vi "Fringe Scan.vi"() -> ()   [LabVIEW 2010]
uses:
  <instrlib>/Keithley 27XX/Public/Data/Read Multiple Direct.vi
  <instrlib>/Keithley 27XX/Keithley 27XX.lvlib
  <vilib>/Analysis/NI_AALBase.lvlib
panel:
  out "Last Value, Volts":dbl
  out "Midpoint":dbl format="%0.3f"
  out "Vpp":dbl
  in  "Integration Time":u16(ring)=10 items=["Slow"=50, "Medium"=10, "Fast"=1]
  out "Waveform Chart":dbl[](graph)
  in  "stop":bool
  in  "VISA resource name":refnum<visa-resource-name>="GPIB0::17::INSTR"
  in  "Serial Configuration (Delicate)":T1={"Baud Rate (9600)"=9600, "Flow Control (1: XON/XOFF)"=1, "Termination Char (0:CR)"=0} {"Termination Char (0:CR)" items=["CR", "LF"]; "Flow Control (1: XON/XOFF)" items=["None", "XON/XOFF", "RTS/CTS (2701 Only)", "XON/XOFF & RTS/CTS (2701 Only)"]; "Baud Rate (9600)" items=["300"=300, "600"=600, "1200"=1200, "2400"=2400, "4800"=4800, "9600"=9600, "19.2k"=19200, "38.4k (2701 Only)"=38400, "57.6k (2701 Only)"=57600, "115.2k (2701 Only)"=115200]}
  # "For use with Keithley 2700, default GPIB address 17"
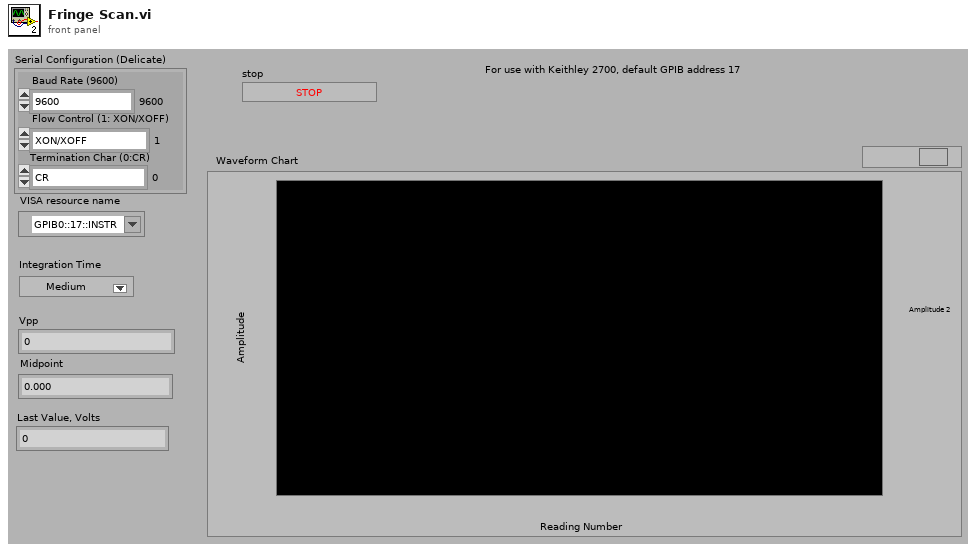
[diagram p1: front panel]
types:
  T1 = cluster{"Baud Rate (9600)":u32, "Flow Control (1: XON/XOFF)":u16, "Termination Char (0:CR)":u16}
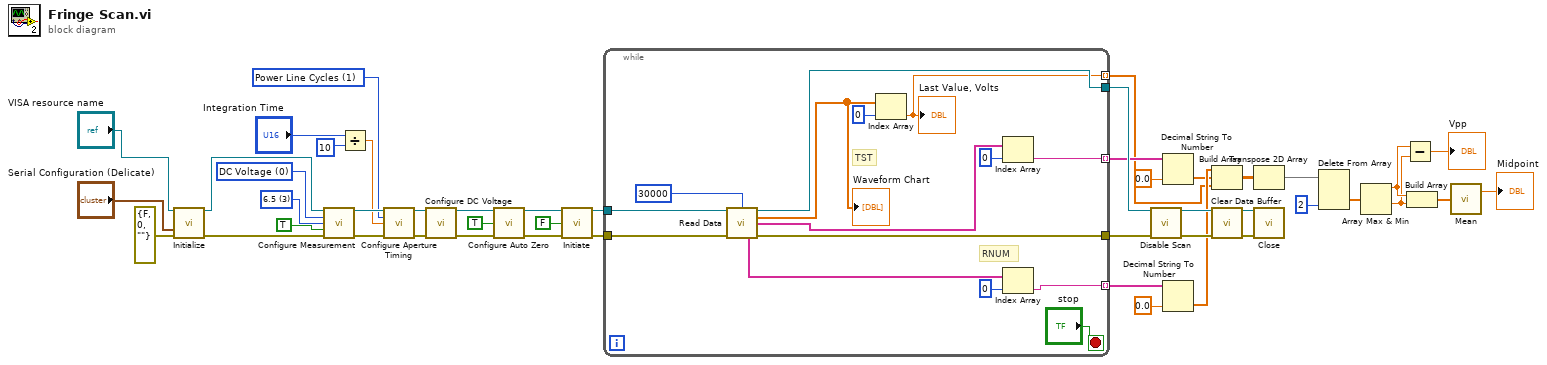
[diagram p0: block diagram]
diagram:
  w32 = u16 1 items=["Seconds", "Power Line Cycles"] ("Timing Units (0: Seconds)")
  w34 = u16 3 items=["3.5", "4.5", "5.5", "6.5"] ("Resolution (3: 6.5 Digits)")
  w35 = u16 0 items=["DC Voltage", "AC Voltage", "DC Current", "AC Current", "Resistance", "Four-Wire Resistance", "Temperature", "Frequency", "Period", "Continuity"] ("Function (0: DC Voltage)")
  n1 = call <instrlib>:"Initialize.vi"("VISA resource name"="VISA resource name", "Serial Configuration"="Serial Configuration (Delicate)", "error in (no error)"=errorcluster {"status"=FALSE, "code"=0, "source"=""}) -> ("VISA resource name out"=w44:refnum<visa-resource-name>, "error out"=w42:errorcluster)  [unwired: 11 in]
  n2 = call <instrlib>:"Configure Measurement.vi"("VISA resource name"=w44, "Function (0: DC Voltage)"=w35, "Resolution (3: 6.5 Digits)"=w34, "Enable Auto Range (True)"=TRUE, "error in (no error)"=w42) -> ("VISA resource name out"=w43:refnum<visa-resource-name>, "error out"=w41:errorcluster)  [unwired: 9 in]
  n3 = Divide(x="Integration Time", y=u16 10) -> (x/y=w28:dbl)
  n4 = call <instrlib>:"Configure Aperture Timing.vi"("VISA resource name"=w43, "Timing Units (0: Seconds)"=w32, "Timing Value (0.020)"=w28, "error in (no error)"=w41) -> ("VISA resource name out"=w39:refnum<visa-resource-name>, "error out"=w38:errorcluster)  [unwired: 10 in]
  n5 = call <instrlib>:"Configure DC Voltage.vi"("VISA resource name"=w39, "error in (no error)"=w38) -> ("VISA resource name out"=w5:refnum<visa-resource-name>, "error out"=w4:errorcluster)  [unwired: 12 in]
  n6 = call <instrlib>:"Configure Auto Zero.vi"("VISA resource name"=w5, "Enable Auto Zero (True)"=TRUE, "error in (no error)"=w4) -> ("VISA resource name out"=w3:refnum<visa-resource-name>, "error out"=w2:errorcluster)  [unwired: 11 in]
  n7 = call <instrlib>:"Initiate.vi"("VISA resource name"=w3, "Enable Continuous Initiation (False)"=FALSE, "error in (no error)"=w2) -> ("VISA resource name out"=w37:refnum<visa-resource-name>, "error out"=w36:errorcluster)  [unwired: 11 in]
  n8 = while {
    tunnel: w37 -> [w60]
    tunnel: w36 -> [w59]
    tunnel: [w53] -> w20 mode=indexing
    tunnel: [w52] -> w21 mode=indexing
    tunnel: [w48] -> w15 mode=indexing
    tunnel: [w50] -> w23
    tunnel: [w49] -> w22
    stop <- "stop" stop-if-true
    # "TST"
    # "RNUM"
    n9 = call-poly <instrlib>:"Read Data.vi"("VISA resource name"=w60, "Timeout (30000 milliseconds)"=u32 30000, "error in (no error)"=w59) -> ("VISA resource name out"=w50:refnum<visa-resource-name>, "Measurement Data"=w47:dbl[], "Time Stamp"=w57:string[], "Reading Number"=w55:string[], "error out"=w49:errorcluster)  [unwired: 7 in, 1 out]
    "Waveform Chart" <- w47
    n10 = Index Array(array=w47, index=0) -> (element=w48:dbl)
    "Last Value, Volts" <- w48
    n11 = Index Array(array=w57, index=0) -> (element=w52:string)
    n12 = Index Array(array=w55, index=0) -> (element=w53:string)
  }
  n13 = call <instrlib>:"Disable Scan.vi"("VISA resource name"=w23, "error in (no error)"=w22) -> ("VISA resource name out"=w27:refnum<visa-resource-name>, "error out"=w26:errorcluster)  [unwired: 12 in]
  n14 = Decimal String To Number(string=w21, default (0L)=0.0 ("default (0 I32)")) -> (number=w16:dbl[])  [unwired: 1 in, 1 out]
  n15 = Decimal String To Number(string=w20, default (0L)=0.0 ("default (0 I32)")) -> (number=w17:dbl[])  [unwired: 1 in, 1 out]
  n16 = Build Array(w17, w16, w15) -> (w14:dbl[][])
  n17 = call <instrlib>:"Clear Data Buffer.vi"("VISA resource name"=w27, "error in (no error)"=w26) -> ("VISA resource name out"=w24:refnum<visa-resource-name>, "error out"=w25:errorcluster)  [unwired: 12 in]
  n18 = Transpose 2D Array(2D array=w14) -> (transposed array=w13:dbl[][])
  n19 = call <instrlib>:"Close.vi"("VISA resource name"=w24, "error in (no error)"=w25) -> ()  [unwired: 13 in, 1 out]
  n20 = Delete From Array(array=w13, index (col)=2 ("disabled index (col)")) -> (deleted portion=w11:dbl[])  [unwired: 2 in, 1 out]
  n21 = Array Max & Min(array=w11) -> (max value=w9:dbl, min value=w8:dbl)  [unwired: 2 out]
  n22 = Subtract(x=w9, y=w8) -> (x-y=→"Vpp":dbl)
  n23 = Build Array(w9, w8) -> (w7:dbl[])
  n24 = call <vilib>:"Mean.vi"("X"=w7) -> ("mean"=→"Midpoint":dbl)  [unwired: 1 out]
